vi "sortPoints.vi"(6 "showComets":bool, 7 "moveCostWeighting":sgl[](array[numeric])=[1.0, 1.0, 1.0], 10 "huntBestStart?":bool, 11 "targetCoords":sgl[][](array[numeric])) -> (1 "sortOrder":i32[](array[numeric]), 3 "sortedCoords":sgl[][](array[numeric]))   [LabVIEW 2022 SP3]
uses:
  <vilib>/Native 3D Graph/xcontrol/3DPC_SurfacePlot.xctl
  Globals/Trav_pos_global.vi
  51c3ce55-73a4-754e-b368-e5b23a609666.vi
panel:
  out "usingUnsorted!":bool
  out "origLength":sgl
  out "sortedLength":sgl
  out "3D Graph":refnum<class "Base Datatype.lvclass">[](xcontrol)
  # "(Right-click and \"Render Window\" to launch resizeable window)"
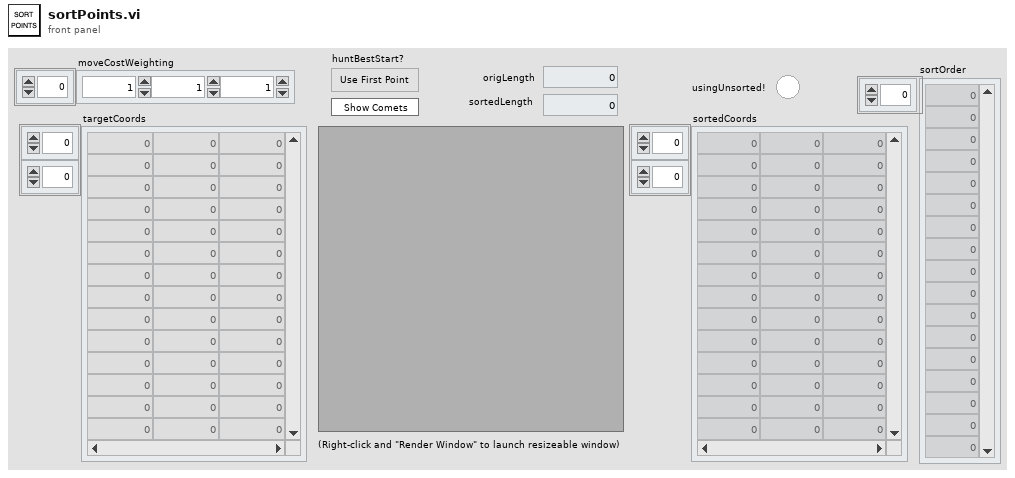
[diagram p1: front panel]
types:
  T1 = typedef "Exclude_cluster.ctl" = cluster{"Sizes":T2, "Name":string, "Exclude Type":T3}
  T2 = typedef "Box_size.ctl" = cluster{"Max":sgl, "Min":sgl}[]
  T3 = typedef "Exclusion_type.ctl" = enum16{"Exclude completely", "Allow only vertical moves"}
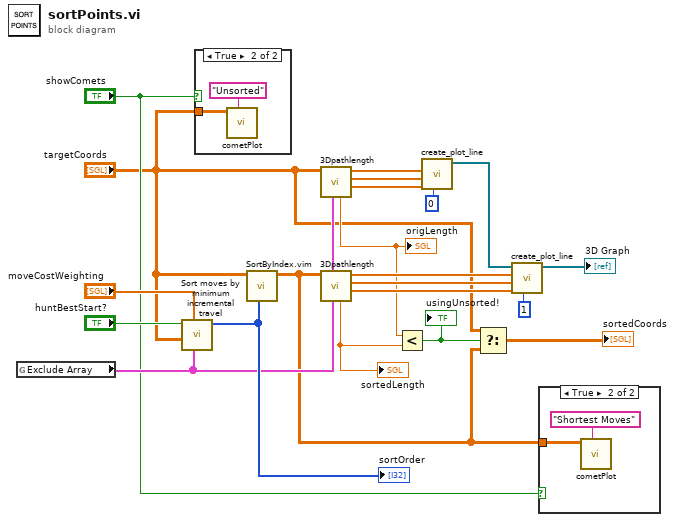
[diagram p0: block diagram]
diagram:
  n1 = global read "Trav_pos_global.vi" "Exclude Array"() -> (w10:T1[])
  n2 = call "Sort moves by minimum incremental travel.vi"("Exclude Array"=w10, "moveCostWeighting"="moveCostWeighting", "Coordinates to move through"="targetCoords", "huntBestStart?"="huntBestStart?") -> ("Order-BestStart"=w11:i32[])  [unwired: 4 in, 3 out]
  "sortOrder" <- w11
  n3 = case shown="True" "showComets" {
    tunnel: "targetCoords" -> [_ w23]
    frame False {
    }
    frame True {
      n4 = call "cometPlot.vi"("sortMethod"="Unsorted", "sortedCoords"=w23) -> ()  [unwired: 9 in, 1 out]
    }
  }
  n5 = call "SortByIndex.vim"("sortOrder"=w11, "2Din"="targetCoords") -> ("2Dout"=w1:sgl[][])  [unwired: 5 in, 1 out]
  n6 = call "3Dpathlength.vi"("Exclude Array"=w10, "targetCoords"="targetCoords") -> ("Zs"=w20:sgl[], "Ys"=w19:sgl[], "Xs"=w18:sgl[], "pathlength"=w5:sgl)  [unwired: 6 in]
  "origLength" <- w5
  n7 = call "3Dpathlength.vi"("Exclude Array"=w10, "targetCoords"=w1) -> ("Zs"=w12:sgl[], "Ys"=w13:sgl[], "Xs"=w14:sgl[], "pathlength"=w6:sgl)  [unwired: 6 in]
  "sortedLength" <- w6
  n8 = Less?(x=w5, y=w6) -> (x < y?=w4:bool)
  "usingUnsorted!" <- w4
  n9 = call <vilib>:"create_plot_line.vi"("plot ID"=0, "z vector"=w20, "y vector"=w19, "x vector"=w18) -> ("plots out"=w17:refnum<class "Base Datatype.lvclass">[])  [unwired: 1 in, 6 out]
  n10 = Select(t="targetCoords", s=w4, f=w1) -> (s? t:f=→"sortedCoords":sgl[][])
  n11 = call <vilib>:"create_plot_line.vi"("plot ID"=1, "z vector"=w12, "y vector"=w13, "x vector"=w14, "plots in"=w17) -> ("plots out"=→"3D Graph":refnum<class "Base Datatype.lvclass">[])  [unwired: 6 out]
  n12 = case shown="True" "showComets" {
    tunnel: w1 -> [_ w25]
    frame False {
    }
    frame True {
      n13 = call "cometPlot.vi"("sortMethod"="Shortest Moves", "sortedCoords"=w25) -> ()  [unwired: 9 in, 1 out]
    }
  }
